vi "_Remote Wait Until Done.vi"(2 "error IO":errorcluster, 3 "Timeout (5s)":dbl=5.0) -> (0 "error out":errorcluster)   [LabVIEW 2015]
uses:
  Type/_RT Command.ctl
  Configuration/_Global Configuration.vi
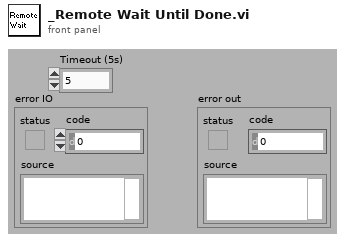
[diagram p1: front panel]
types:
  T1 = typedef "_RT Command.ctl" = enum16{"Start", "Stop", "Runtime Update", "Get Data", "Get Info", "Get Status", "Get Param", "Get Config", "Get Table", "Read ADC", "Set Oscillator", "Update Config", "Update Table", "Set All Pol", "Set Pol and DC", "Set Max Mass", "Toggle RP", "Toggle EL", "Set PIC", "Initialize Turbo", "Send Turbo Comm", "Close Turbo", "P1", "P2", "P3", "Send Serial", "Set LC Out", "Get LC In", "Read VAC", "Test Table", "Toggle Power", "Get Startup", "Set Startup", "Get ADC Table", "Set ADC Table", "Get Brief Status", "Get Detail Status", "Auxiliary Update", "Set CC Logics", "Set CC Input Logics", "Ignore Error"}
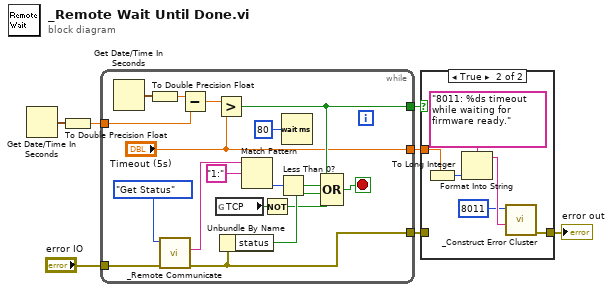
[diagram p0: block diagram]
diagram:
  n1 = Get Date/Time In Seconds() -> (seconds since 1Jan1904=w6:timestamp)
  n2 = To Double Precision Float(number=w6) -> (double precision float=w5:dbl)
  n3 = while {
    tunnel: "error IO" -> [w24]
    tunnel: [w11] -> w4
    tunnel: w5 -> [w19]
    tunnel: [w14] -> w2
    tunnel: ["Timeout (5s)"] -> w1
    stop <- w15 stop-if-true
    n4 = Get Date/Time In Seconds() -> (seconds since 1Jan1904=w21:timestamp)
    n5 = To Double Precision Float(number=w21) -> (double precision float=w20:dbl)
    n6 = call "_Remote Communicate.vi"("error in (no error)"=w24, "Command"=_RT_Command."Get Status") -> ("error out"=w11:errorcluster, "Info"=w10:string)  [unwired: 4 in, 2 out]
    n7 = Subtract(x=w20, y=w19) -> (x-y=w18:dbl)
    n8 = Greater?(x=w18, y="Timeout (5s)") -> (0:w14:bool)
    n9 = global read "_Global Configuration.vi" "TCP"() -> (w9:bool)
    n10 = Unbundle By Name(w11) -> ("status"=w16:bool)
    n11 = Match Pattern(string=w10, regular expression="1:") -> (offset past match=w22:i32)  [unwired: 4 out]
    n12 = Not(x=w9) -> (.not. x?=w8:bool)
    n13 = Less Than 0?(x=w22) -> (x < 0?=w17:bool)
    n14 = Wait (ms)(milliseconds to wait=u32 80) -> ()  [unwired: 1 out]
    n15 = Compound Arithmetic op=OR(w14, w17, w16, w8) -> (w15:bool)
  }
  n16 = case shown="True" w2 {
    tunnel: w4 -> [w26 _]
    tunnel: [w26 w32] -> w3
    tunnel: w1 -> [_ w31]
    frame False {
    }
    frame True {
      n17 = To Long Integer(number=w31) -> (32bit integer=w30:i32)
      n18 = Format Into String(format string="8011: %ds timeout while waiting for firmware ready.", w30) -> (resulting string=w28:string)  [unwired: 2 in, 1 out]
      n19 = call "_Construct Error Cluster.vi"("reason"=w28, "errorCode"=8011) -> ("error out"=w32:errorcluster)  [unwired: 2 in, 3 out]
    }
  }
  "error out" <- w3
